vi "destroy.vi"(8 "error in":errorcluster, 11 "event reporter in":refnum<class "event reporter.lvclass">) -> (0 "error out":errorcluster)   [LabVIEW 2013, in "event reporter.lvclass"]
uses:
  event reporter.lvclass
  event reporter.lvclass/event reporter.ctl
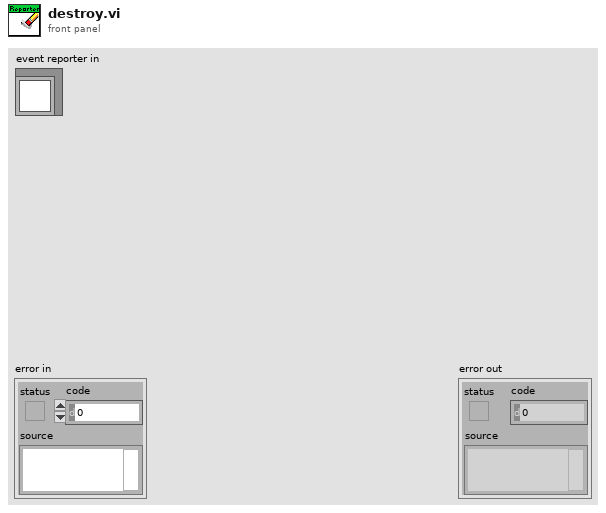
[diagram p1: front panel]
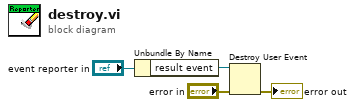
[diagram p0: block diagram]
diagram:
  n1 = Unbundle By Name("event reporter in") -> ("result event"=w1:refnum<user-event>)
  n2 = Destroy User Event(user event=w1, error in="error in") -> (error out=→"error out":errorcluster)
